vi "resultsColumnsBasic.vi"() -> (2 "chValues":string[](array[string]), 3 "chNames":string[](array[string]))   [LabVIEW 2021]
uses:
  Globals/Meas_global.vi
  Globals/Trav_pos_global.vi
  Globals/Preference_global.vi
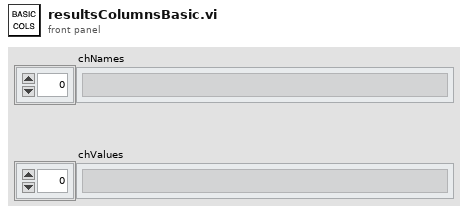
[diagram p1: front panel]
types:
  T1 = typedef "Post_Process.ctl" = enum16{"Take New Data", "Post Process Raw Data File"}
  T2 = typedef "Analysis_info_cluster.ctl" = cluster{"Colour":u32, "Inst type":T3, "Inst name":string, "Symbol":string, "Code name":string, "Extra Info":string, "Inst Array":T4, "Extra Titles":string[], "Extra Values":string[], "U":dbl, "u^2":dbl, "u^3":dbl, "u^4":dbl, "Skew_u":dbl, "Kurt_u":dbl, "Sd Error in Mean":dbl, "% u'/U":dbl, "X":dbl, "Y":dbl, "Z":dbl, "Timescale integral Estimate":dbl, "Sd Error in Variance":dbl, "Calib File":path, "Calib Constants":dbl[], "Output Position":bool, "Stats":enum16{"None", "Basic", "Full"}, "Av Sampling Rate":dbl, "Av No of Samples":dbl, "Total Meas Time (s)":dbl, "ADAM Ch Name":string, "Max value":dbl, "Min value":dbl, "Req Sample Rate Hz":dbl, "Sync Delay Time (s)":dbl, "Ch No":i16, "Device":string, "Use Latest Calib":bool, "Port":string, "Metadata Ch Names":string[], "Metadata Ch Values":string[], "Label":string}
  T3 = typedef "Inst_type.ctl" = enum16{"Raw voltage", "Raw with zero offsetting", "Propeller anemometer", "Pressure Transducer", "Pitot-static tube", "Hot wire", "Cross wire 1", "Cross wire 2", "Generic Linear", "Generic Polynomial", "Generic BackPoly", "Fast FID", "Thermocouple", "Cold wire", "Pulsed Wire", "LDA Vel", "LDA Tran time", "LDA Arr time", "Microphone"}
  T4 = typedef "Instrument_Array.ctl" = enum16{"PWA", "LDA", "Analogue"}
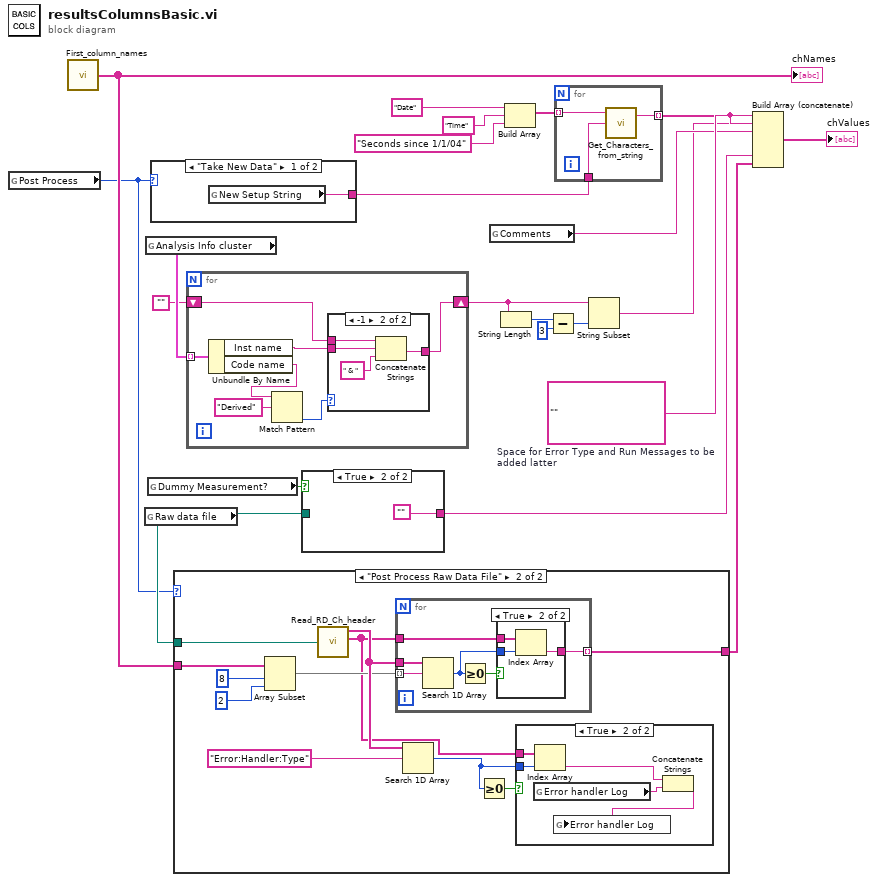
[diagram p0: block diagram]
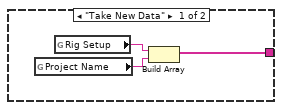
[diagram p2: hidden frame]
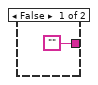
[diagram p4: hidden frame]
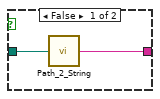
[diagram p5: hidden frame]
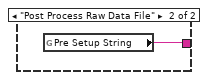
[diagram p7: hidden frame]
diagram:
  w16 = ""  # Space for Error Type and Run Messages to be added latter
  n1 = global read "Meas_global.vi" "Post Process"() -> (w20:T1)
  n2 = call "First_column_names.vi"() -> ("Array"=w22:string[])
  "chNames" <- w22
  n3 = global read "Meas_global.vi" "Raw data file"() -> (w21:path)
  n4 = global read "Meas_global.vi" "Analysis Info cluster"() -> (w19:T2[])
  n5 = global read "Trav_pos_global.vi" "Dummy Measurement?"() -> (w18:bool)
  n6 = case shown="\"Take New Data\"" w20 {
    tunnel: [w23 w24] -> w6
    frame "Take New Data" {
      n7 = global read "Meas_global.vi" "New Setup String"() -> (w23:string)
    }
    frame "Post Process Raw Data File" {
      n8 = global read "Meas_global.vi" "Pre Setup String"() -> (w24:string)
    }
  }
  n9 = case shown="\"Post Process Raw Data File\"" w20 {
    tunnel: w22 -> [_ w38]
    tunnel: w21 -> [_ w35]
    tunnel: [w27 w34] -> w17
    frame "Take New Data" {
      n10 = global read "Preference_global.vi" "Project Name"() -> (w26:string)
      n11 = global read "Preference_global.vi" "Rig Setup"() -> (w25:string)
      n12 = Build Array(w25, w26) -> (w27:string[])
    }
    frame "Post Process Raw Data File" {
      n13 = Array Subset(array=w38, index=8, length=2) -> (w29:string[])
      n14 = call "Read_RD_Ch_header.vi"("Raw data file"=w35) -> ("Ch Name Out"=w33:string[], "Ch Values"=w28:string[])  [unwired: 2 out]
      n15 = for {
        tunnel: w33 -> [w49]
        tunnel: w28 -> [w46]
        tunnel: [w45] -> w34 mode=indexing
        tunnel: w29 -> [w44] mode=indexing
        n16 = Search 1D Array(1D array=w49, element=w44) -> (index of element=w47:i32)  [unwired: 1 out]
        n17 = Greater Or Equal To 0?(x=w47) -> (x >= 0?=w48:bool)
        n18 = case shown="True" w48 {
          tunnel: w47 -> [_ w53]
          tunnel: w46 -> [_ w52]
          tunnel: ["" w51] -> w45
          frame False {
          }
          frame True {
            n19 = Index Array(array=w52, index=w53) -> (element=w51:string)
          }
        }
      }
      n20 = Search 1D Array(1D array=w33, element="Error:Handler:Type") -> (index of element=w30:i32)  [unwired: 1 out]
      n21 = Greater Or Equal To 0?(x=w30) -> (x >= 0?=w31:bool)
      n22 = case shown="True" w31 {
        tunnel: w30 -> [_ w43]
        tunnel: w28 -> [_ w42]
        frame False {
        }
        frame True {
          n23 = global read "Meas_global.vi" "Error handler Log"() -> (w41:string)
          n24 = Index Array(array=w42, index=w43) -> (element=w40:string)
          n25 = Concatenate Strings(w40, w41) -> (w39:string)
          n26 = global write "Meas_global.vi" "Error handler Log"(w39) -> ()
        }
      }
    }
  }
  n27 = for {
    shift-right: [w59] -> w10
    shift-left: "" -> [w60]
    tunnel: w19 -> [w58] mode=indexing
    n28 = Unbundle By Name(w58) -> ("Inst name"=w57:string, "Code name"=w56:string)
    n29 = Match Pattern(string=w56, regular expression="Derived") -> (offset past match=w54:i32)  [unwired: 1 in, 3 out]
    n30 = case shown="-1" w54 {
      tunnel: w60 -> [w61 w65]
      tunnel: [w61 w64] -> w59
      tunnel: w57 -> [_ w62]
      frame 0, Default {
      }
      frame -1 {
        n31 = Concatenate Strings(w65, w62, " & ") -> (w64:string)
      }
    }
  }
  n32 = case shown="True" w18 {
    tunnel: [w67 ""] -> w15
    tunnel: w21 -> [w66 _]
    frame False {
      n33 = call "Path_2_String.vi"("Real Path"=w66) -> ("Path String"=w67:string)
    }
    frame True {
    }
  }
  n34 = global read "Meas_global.vi" "Comments"() -> (w13:string)
  n35 = String Length(string=w10) -> (length=w7:i32)
  n36 = Build Array("Date", "Time", "Seconds since 1/1/04") -> (w4:string[])
  n37 = Subtract(x=w7, y=3) -> (x-y=w9:i32)
  n38 = for {
    tunnel: w4 -> [w71] mode=indexing
    tunnel: w6 -> [w70]
    tunnel: [w69] -> w5 mode=indexing
    n39 = call "Get_Characters_from_string.vi"("Input string"=w70, "Variable name"=w71) -> ("Value"=w69:string)  [unwired: 1 in, 1 out]
  }
  n40 = String Subset(string=w10, length (rest)=w9) -> (substring=w12:string)  [unwired: 1 out]
  n41 = Build Array (concatenate)(w5, w12, w13, w16, w16, w15, w17) -> (→"chValues":string[])
